vi "Configuracao.Leitura.vi"(8 "error in":errorcluster) -> (0 "error out":errorcluster)   [LabVIEW 2019]
uses:
  <vilib>/Utility/xml.llb/Read From XML File(string).vi
  Configuracao.Variaveis.vi
  TelaParametrosTeste/VariaveisParametros.vi
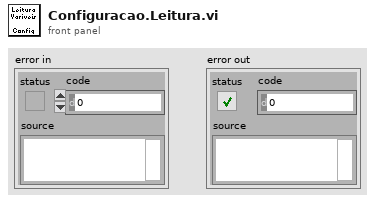
[diagram p1: front panel]
types:
  T1 = cluster{"Texpontos senoide":string, "PicoRotacaoMax":dbl, "PicoRotacaoMin":dbl, "RotacoesMinuto":dbl, "TaxaGeracao":dbl}
  T2 = cluster{"TempRampas":dbl, "PicoMax":dbl, "TextUnidMed":string}
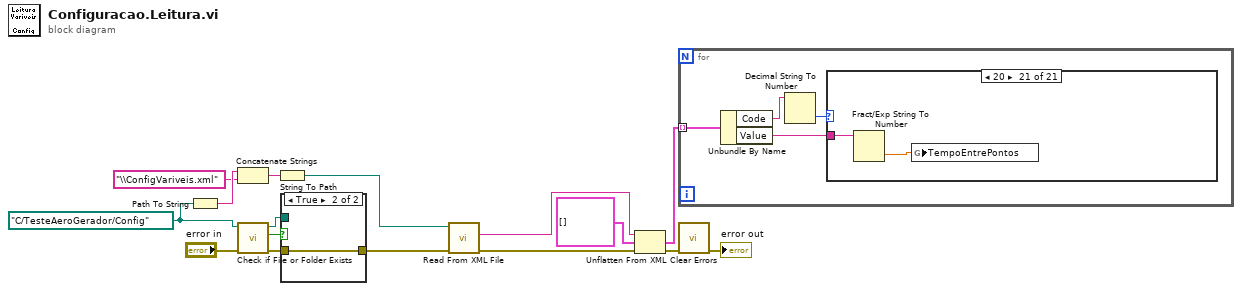
[diagram p0: block diagram]
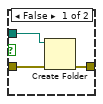
[diagram p2: hidden frame]
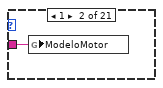
[diagram p4: hidden frame]
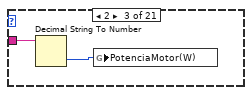
[diagram p5: hidden frame]
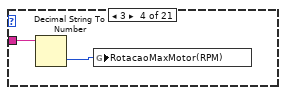
[diagram p6: hidden frame]
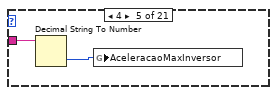
[diagram p7: hidden frame]
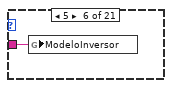
[diagram p8: hidden frame]
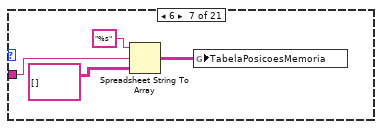
[diagram p9: hidden frame]
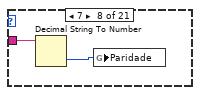
[diagram p10: hidden frame]
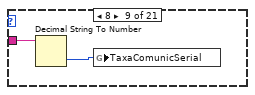
[diagram p11: hidden frame]
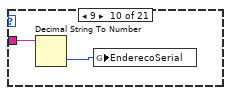
[diagram p12: hidden frame]
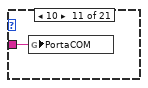
[diagram p13: hidden frame]
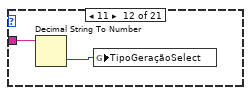
[diagram p14: hidden frame]
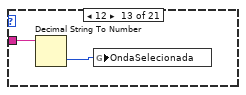
[diagram p15: hidden frame]
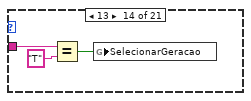
[diagram p16: hidden frame]
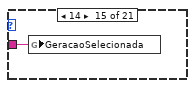
[diagram p17: hidden frame]
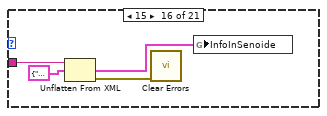
[diagram p18: hidden frame]
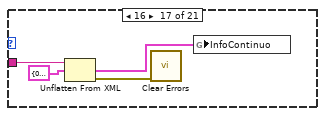
[diagram p19: hidden frame]
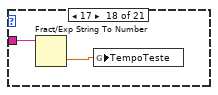
[diagram p20: hidden frame]
diagram:
  w10 = path "C:/TesteAeroGerador/Config" ("XML File Path")
  n1 = Path To String(path=w10) -> (string=w9:string)
  n2 = Concatenate Strings(w9, "\\ConfigVariveis.xml") -> (w7:string)
  n3 = call <vilib>:"Check if File or Folder Exists.vi"("error in (no error)"="error in", "path"=w10) -> ("error out"=w11:errorcluster, "file or folder exists?"=w12:bool, "dup path"=w6:path)  [unwired: 7 in]
  n4 = String To Path(string=w7) -> (path=w4:path)
  n5 = case shown="True" w12 {
    tunnel: w6 -> [w19 _]
    tunnel: w11 -> [w18 w20]
    tunnel: [w17 w20] -> w5
    frame False {
      n6 = Create Folder(path (use dialog)=w19, error in=w18) -> (error out=w17:errorcluster)  [unwired: 1 in, 2 out]
    }
    frame True {
    }
  }
  n7 = call-poly <vilib>:"Read From XML File.vi"("error in (no error)"=w5, "XML File Path"=w4) -> ("error out"=w2:errorcluster, "XML Elements"=w1:string)  [unwired: 7 in, 1 out]
  n8 = Unflatten From XML(xml string=w1, type=cluster{"Code":string, "Value":string}[] [] ("anything"), error in (no error)=w2) -> (value=w15:cluster{"Code":string, "Value":string}[], error out=w14:errorcluster)
  n9 = for {
    tunnel: w15 -> [w24] mode=indexing
    n10 = Unbundle By Name(w24) -> ("Code"=w23:string, "Value"=w21:string)
    n11 = Decimal String To Number(string=w23) -> (number=w22:i32)  [unwired: 2 in, 1 out]
    n12 = case shown="20" w22 {
      tunnel: w21 -> [_ w25 w27 w29 w31 w32 w33 w38 w40 w42 w43 w44 w46 w50 w51 w53 w58 w61 w63 w68 w71]
      frame 0, Default {
      }
      frame 1 {
        n13 = global write "Configuracao.Variaveis.vi" "ModeloMotor"(w25) -> ()
      }
      frame 2 {
        n14 = Decimal String To Number(string=w27) -> (number=w26:i32)  [unwired: 2 in, 1 out]
        n15 = global write "Configuracao.Variaveis.vi" "PotenciaMotor(W)"(w26) -> ()
      }
      frame 3 {
        n16 = Decimal String To Number(string=w29) -> (number=w28:i32)  [unwired: 2 in, 1 out]
        n17 = global write "Configuracao.Variaveis.vi" "RotacaoMaxMotor(RPM)"(w28) -> ()
      }
      frame 4 {
        n18 = Decimal String To Number(string=w31) -> (number=w30:i32)  [unwired: 2 in, 1 out]
        n19 = global write "Configuracao.Variaveis.vi" "AceleracaoMaxInversor"(w30) -> ()
      }
      frame 5 {
        n20 = global write "Configuracao.Variaveis.vi" "ModeloInversor"(w32) -> ()
      }
      frame 6 {
        n21 = Spreadsheet String To Array(format string="%s", spreadsheet string=w33, array type (2D Dbl)=string[][] []) -> (array=w34:string[][])  [unwired: 1 in]
        n22 = global write "Configuracao.Variaveis.vi" "TabelaPosicoesMemoria"(w34) -> ()
      }
      frame 7 {
        n23 = Decimal String To Number(string=w38) -> (number=w37:i32)  [unwired: 2 in, 1 out]
        n24 = global write "Configuracao.Variaveis.vi" "Paridade"(w37) -> ()
      }
      frame 8 {
        n25 = Decimal String To Number(string=w40) -> (number=w39:i32)  [unwired: 2 in, 1 out]
        n26 = global write "Configuracao.Variaveis.vi" "TaxaComunicSerial"(w39) -> ()
      }
      frame 9 {
        n27 = Decimal String To Number(string=w42) -> (number=w41:i32)  [unwired: 2 in, 1 out]
        n28 = global write "Configuracao.Variaveis.vi" "EnderecoSerial"(w41) -> ()
      }
      frame 10 {
        n29 = global write "Configuracao.Variaveis.vi" "PortaCOM"(w43) -> ()
      }
      frame 11 {
        n30 = Decimal String To Number(string=w44) -> (number=w45:i32)  [unwired: 2 in, 1 out]
        n31 = global write "VariaveisParametros.vi" "TipoGeraçãoSelect"(w45) -> ()
      }
      frame 12 {
        n32 = Decimal String To Number(string=w46) -> (number=w47:i32)  [unwired: 2 in, 1 out]
        n33 = global write "VariaveisParametros.vi" "OndaSelecionada"(w47) -> ()
      }
      frame 13 {
        n34 = Equal?(x=w50, y="T") -> (x = y?=w48:bool)
        n35 = global write "VariaveisParametros.vi" "SelecionarGeracao"(w48) -> ()
      }
      frame 14 {
        n36 = global write "VariaveisParametros.vi" "GeracaoSelecionada"(w51) -> ()
      }
      frame 15 {
        n37 = Unflatten From XML(xml string=w53, type=T1 {"Texpontos senoide"="O máximo é 60 pontos por minuto", "PicoRotacaoMax"=0.0, "PicoRotacaoMin"=0.0, "RotacoesMinuto"=0.0, "TaxaGeracao"=0.0} ("InfoInSenoide")) -> (value=w52:T1, error out=w55:errorcluster)  [unwired: 1 in]
        n38 = call <vilib>:"Clear Errors.vi"("error in (no error)"=w55) -> ()  [unwired: 5 in, 2 out]
        n39 = global write "VariaveisParametros.vi" "InfoInSenoide"(w52) -> ()
      }
      frame 16 {
        n40 = Unflatten From XML(xml string=w58, type=T2 {"TempRampas"=0.0, "PicoMax"=0.0, "TextUnidMed"="segundos"} ("InfoContinuo")) -> (value=w56:T2, error out=w59:errorcluster)  [unwired: 1 in]
        n41 = call <vilib>:"Clear Errors.vi"("error in (no error)"=w59) -> ()  [unwired: 5 in, 2 out]
        n42 = global write "VariaveisParametros.vi" "InfoContinuo"(w56) -> ()
      }
      frame 17 {
        n43 = Fract/Exp String To Number(string=w61) -> (number=w60:dbl)  [unwired: 3 in, 1 out]
        n44 = global write "VariaveisParametros.vi" "TempoTeste"(w60) -> ()
      }
      frame 18 {
        n45 = Spreadsheet String To Array(format string="%s", spreadsheet string=w63, array type (2D Dbl)=string[][] []) -> (array=w62:string[][])  [unwired: 1 in]
        n46 = global write "VariaveisParametros.vi" "ListaMedicaoPorta"(w62) -> ()
      }
      frame 19 {
        n47 = Spreadsheet String To Array(format string="%s", spreadsheet string=w68, array type (2D Dbl)=string[] []) -> (array=w67:string[])  [unwired: 1 in]
        n48 = Fract/Exp String To Number(string=w67) -> (number=w66:dbl[])  [unwired: 3 in, 1 out]
        n49 = global write "VariaveisParametros.vi" "Pontos"(w66) -> ()
      }
      frame 20 {
        n50 = Fract/Exp String To Number(string=w71) -> (number=w72:dbl)  [unwired: 3 in, 1 out]
        n51 = global write "VariaveisParametros.vi" "TempoEntrePontos"(w72) -> ()
      }
    }
  }
  n52 = call <vilib>:"Clear Errors.vi"("error in (no error)"=w14) -> ("error out"=→"error out":errorcluster)  [unwired: 5 in, 1 out]
